vi "Open Customized Ini Tokens Folder.vi"   [LabVIEW 2017, in "NEVSTOP_QuickDrop.lvlib"]
doc: "Opens the folder that holds the customized LabVIEW.ini token files in a Windows Explorer window."
uses:
  NEVSTOP_QuickDrop.lvlib
  QD_Smart Open VI Location/Smart Open VI Location.lvlib
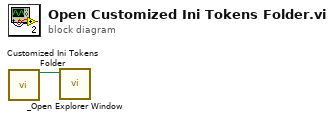
[diagram p0: block diagram]
diagram:
  n1 = call "Customized Ini Tokens Folder.vi"() -> ("appended path"=w1:path)  [unwired: 19 in]
  n2 = call "_Open Explorer Window.vi"("Directory or File"=w1) -> ()  [unwired: 10 in, 1 out]
